vi "时序检查.vi"(8 "时序优先":bool, 10 "nplc":dbl, 11 "测量间隔":dbl) -> (2 "nplc输出":dbl, 3 "测量间隔输出":dbl)   [LabVIEW 2020, in "功能选择.xctl"]
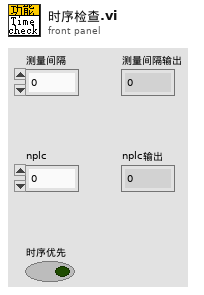
[diagram p1: front panel]
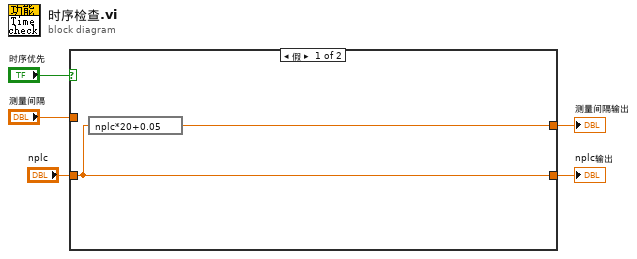
[diagram p0: block diagram]
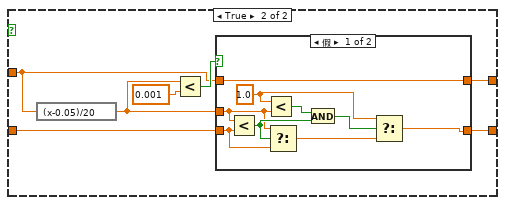
[diagram p2: hidden frame]
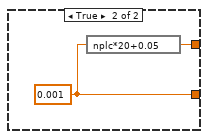
[diagram p3: hidden frame]
diagram:
  n1 = case shown="假" "时序优先" {
    tunnel: "测量间隔" -> [_ w9]
    tunnel: "nplc" -> [w6 w14]
    tunnel: [w7 w8] -> w3
    tunnel: [w6 w13] -> w2
    frame False {
      n2 = expression code="nplc*20+0.05"(w6) -> (w7:dbl)
    }
    frame True {
      n3 = expression code="(x-0.05)/20"(w9) -> (w11:dbl)
      n4 = Less?(x=w11, y=0.001) -> (x < y?=w12:bool)
      n5 = case shown="假" w12 {
        tunnel: w14 -> [w23 _]
        tunnel: [w19 w25] -> w13
        tunnel: w11 -> [w17 _]
        tunnel: w9 -> [w15 _]
        tunnel: [w15 w24] -> w8
        frame False {
          w18 = 1.0 ("t")
          n6 = Less?(x=w17, y=w23) -> (x < y?=w22:bool)
          n7 = Less?(x=w18, y=w17) -> (x < y?=w16:bool)
          n8 = Select(t=w17, s=w22, f=w23) -> (s? t:f=w20:dbl)
          n9 = And(x=w16, y=w22) -> (x .and. y?=w21:bool)
          n10 = Select(t=w18, s=w21, f=w20) -> (s? t:f=w19:dbl)
        }
        frame True {
          w25 = 0.001 ("nplc")
          n11 = expression code="nplc*20+0.05"(w25) -> (w24:dbl)
        }
      }
    }
  }
  "测量间隔输出" <- w3
  "nplc输出" <- w2
